vi "Excel_Read_XLSX.vi"(8 "error in (no error)":errorcluster, 10 "Truncate? (T)":bool=TRUE, 11 "Path in (xlsx,tsv,txt,csv,xml)":path) -> (0 "error out":errorcluster, 2 "Worksheets":T1(array[cluster]), 3 "Path out":path)   [LabVIEW 2018]
uses:
  <vilib>/zip/NI_Unzip.lvlib
  <vilib>/ErrorRing/Error Ring.xnode
  <vilib>/Utility/error.llb/Error Cluster From Error Code.vi
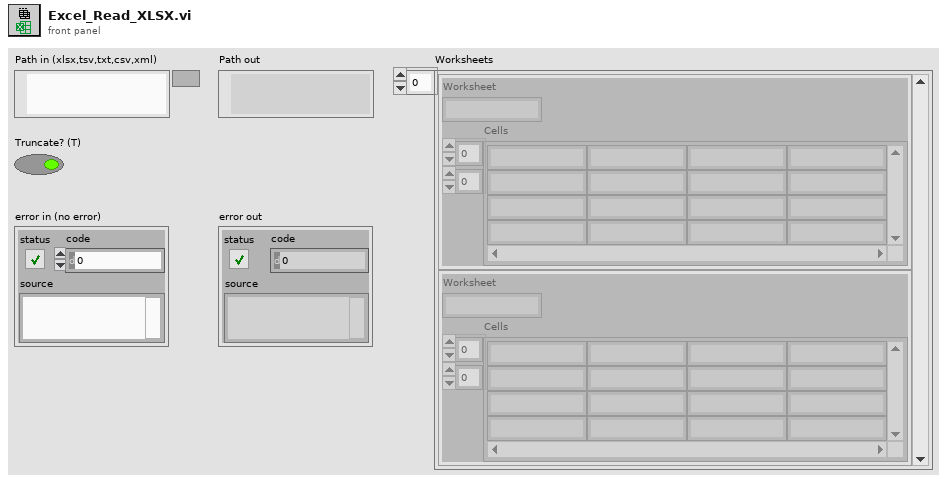
[diagram p1: front panel]
types:
  T1 = cluster{"Worksheet":string, "Cells":string[][]}[]
  T2 = cluster{"path":path, "sharedStrings.xml":string, "workbook.xml":string, "worksheet.xml":string[], "worksheet.xml IDs":i32[], "sharedStrings":string[], "SheetIDs":i32[], "Worksheets":cluster{"Worksheet":string, "Cells":string[][]}[], "sheetData":string[]}
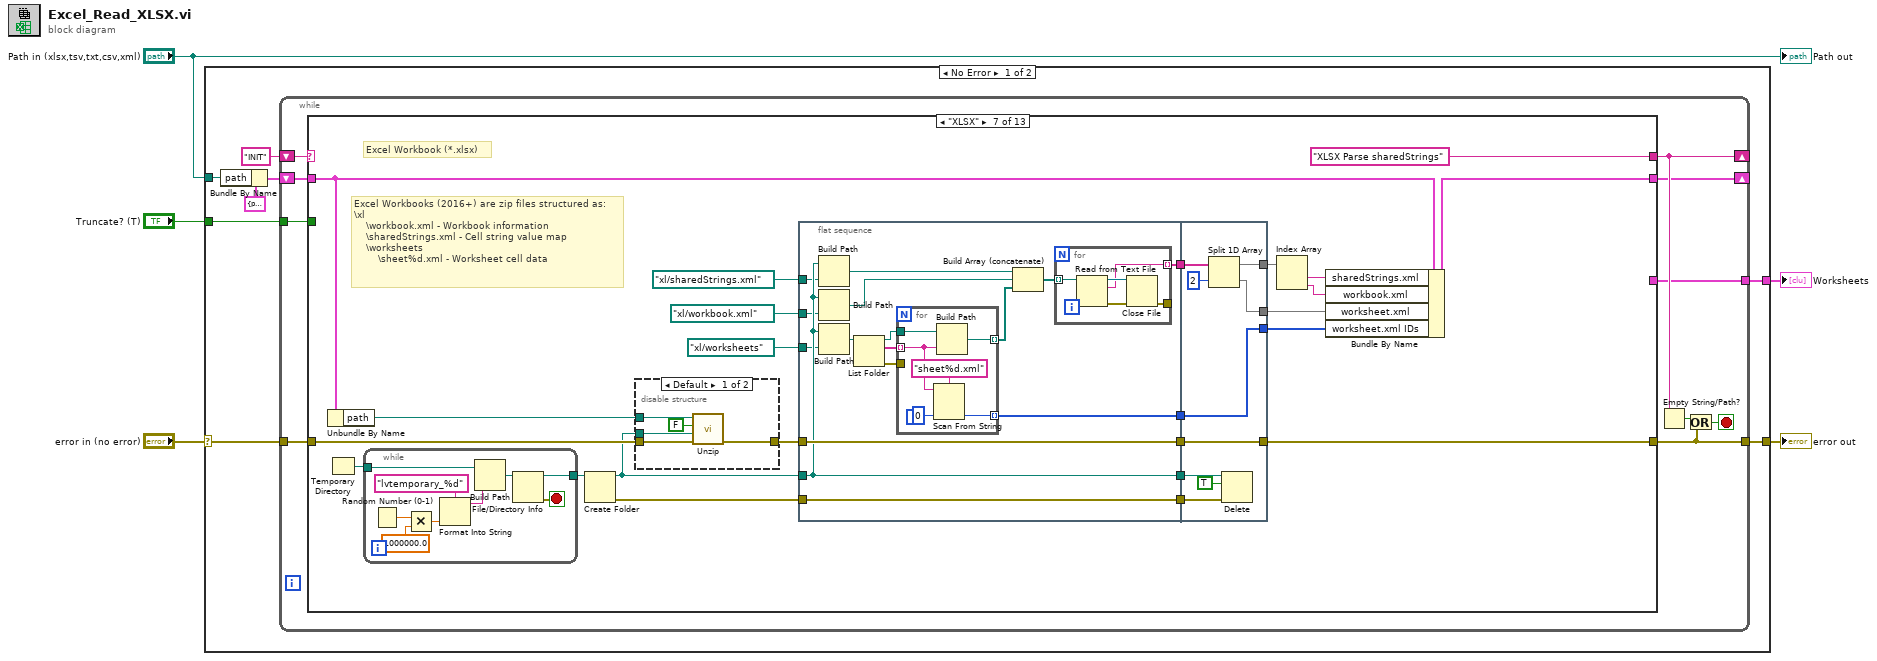
[diagram p0: block diagram]
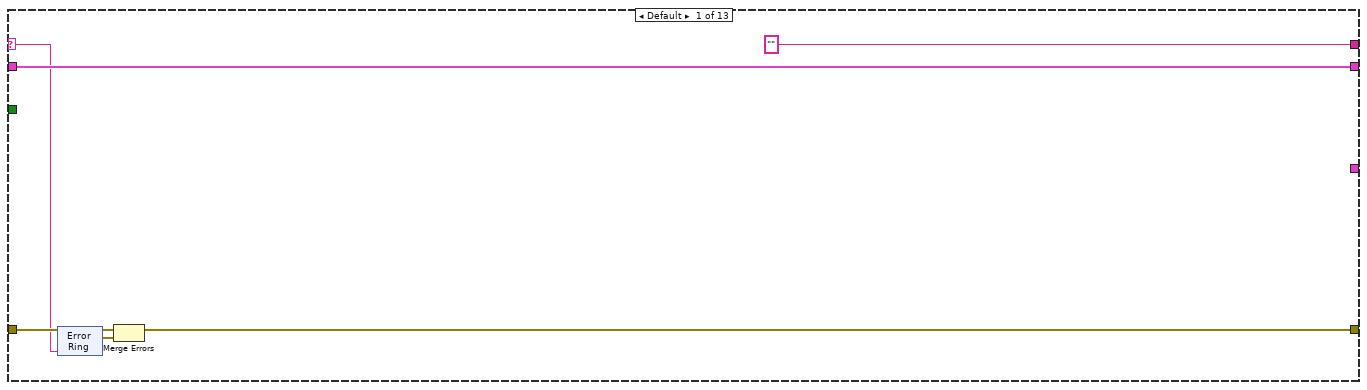
[diagram p2: hidden frame]
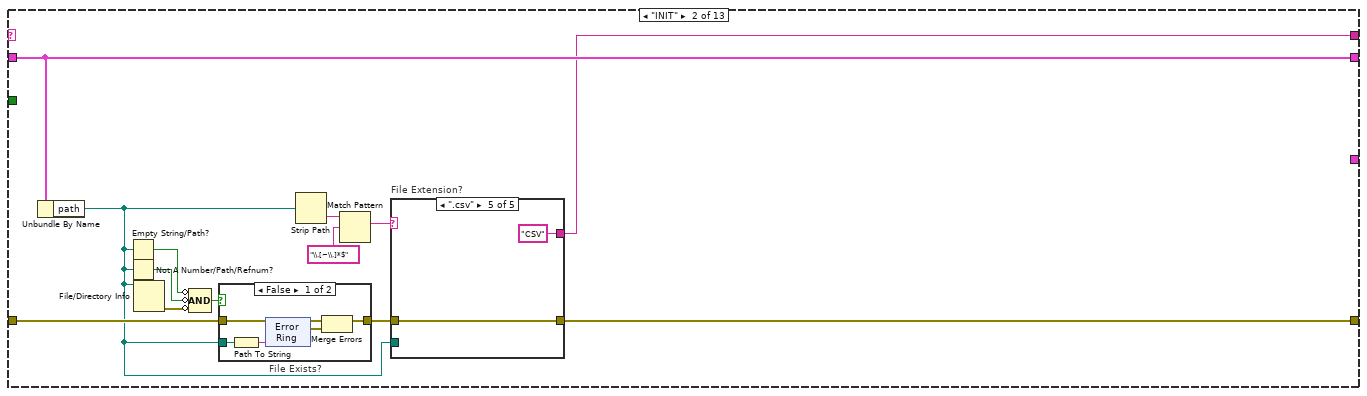
[diagram p3: hidden frame]
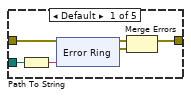
[diagram p4: hidden frame]
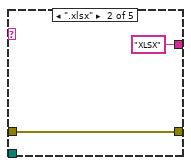
[diagram p5: hidden frame]
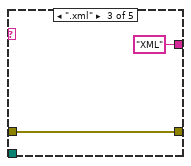
[diagram p6: hidden frame]
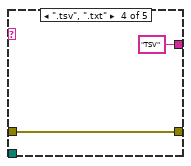
[diagram p7: hidden frame]
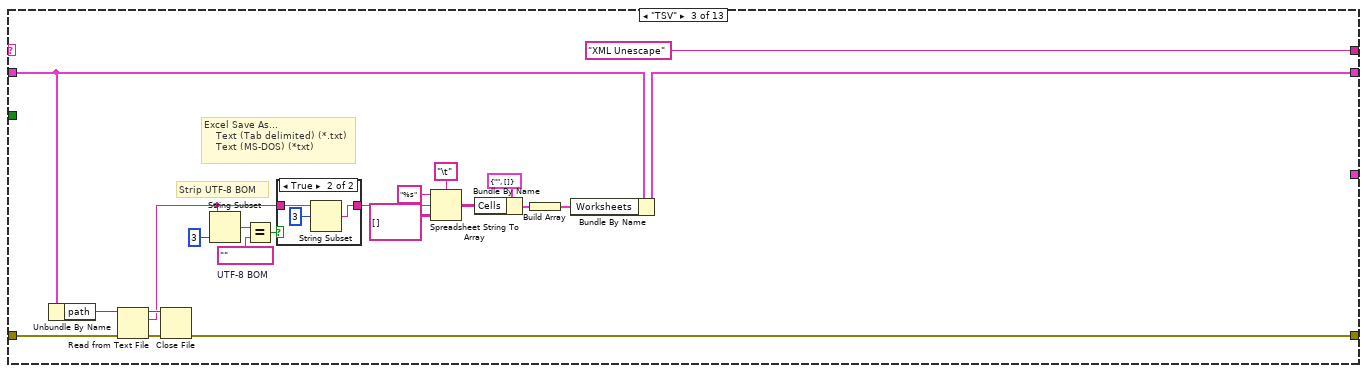
[diagram p9: hidden frame]
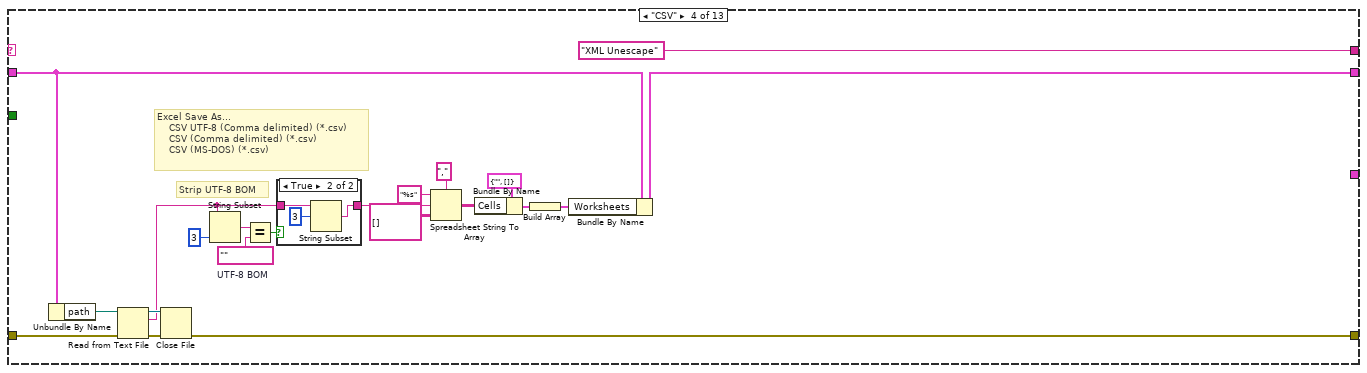
[diagram p11: hidden frame]
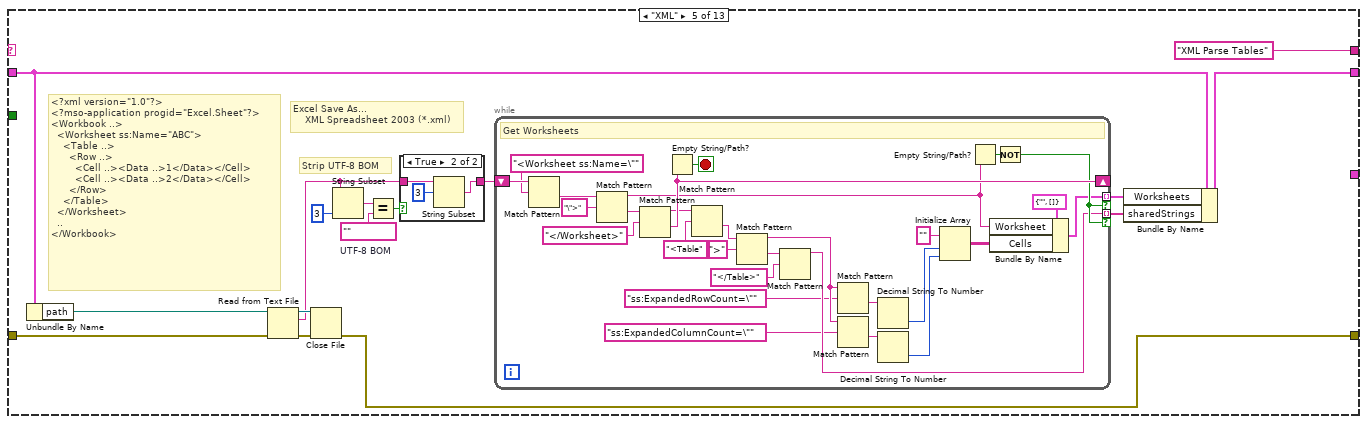
[diagram p13: hidden frame]
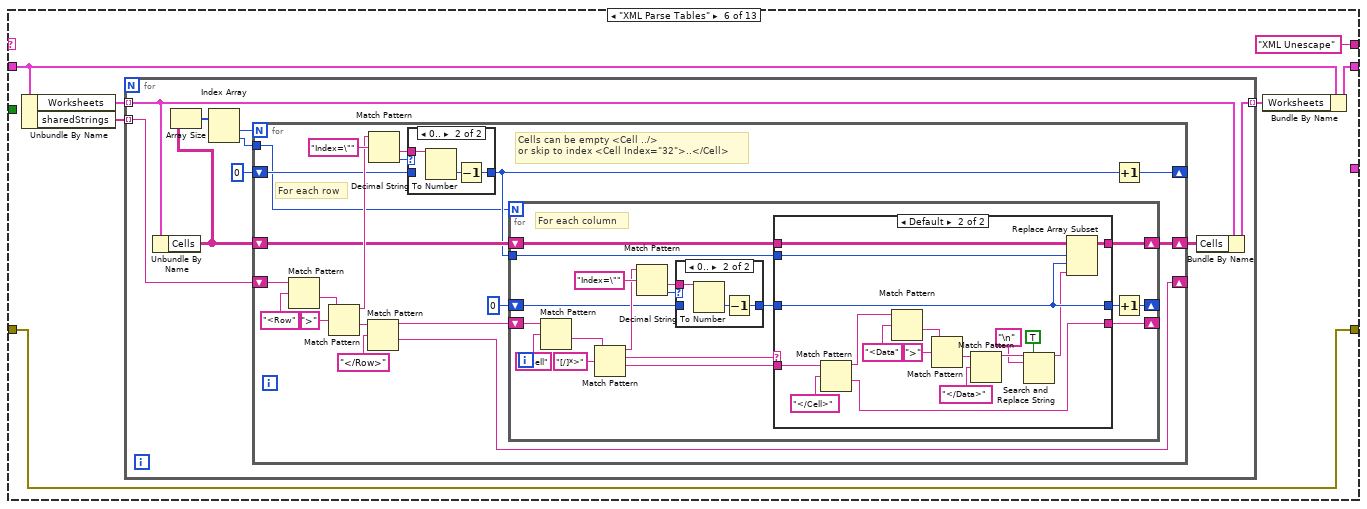
[diagram p15: hidden frame]
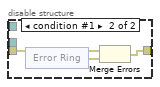
[diagram p19: hidden frame]
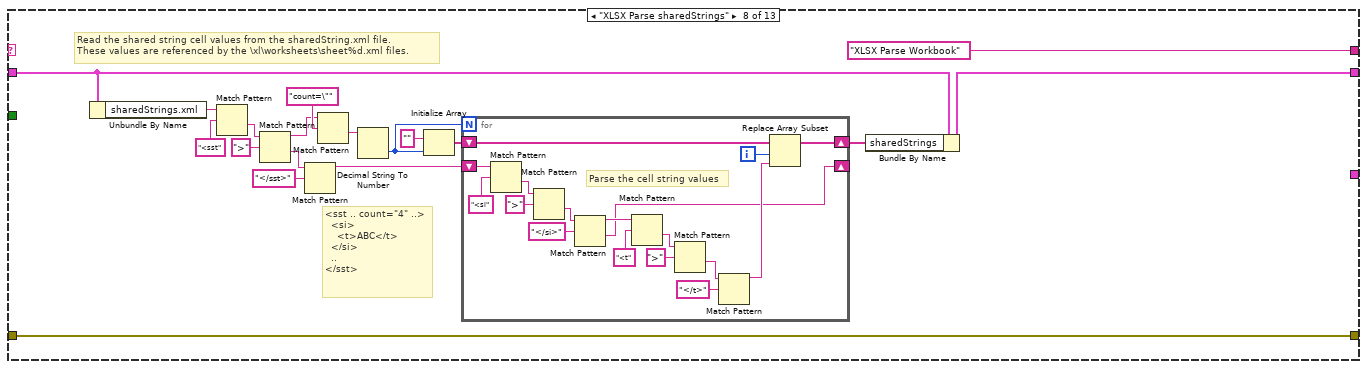
[diagram p20: hidden frame]
diagram:
  n1 = case shown="No Error" "error in (no error)" {
    selector: "error in (no error)" -> [w12 w624]
    tunnel: "Path in (xlsx,tsv,txt,csv,xml)" -> [w9 _]
    tunnel: [w8 w624] -> w3
    tunnel: [w7 _] -> w2
    tunnel: "Truncate? (T)" -> [w6 _]
    frame No Error {
      n2 = Bundle By Name(cluster=T2 {"path"=path "", "sharedStrings.xml"="", "workbook.xml"="", "worksheet.xml"=[], "worksheet.xml IDs"=[], "sharedStrings"=[], "SheetIDs"=[], "Worksheets"=[], "sheetData"=[]} ("StateData"), "path"=w9) -> (w10:T2)
      n3 = while {
        shift-right: [w18] -> _
        shift-left: "INIT" -> [w23]
        tunnel: w12 -> [w22]
        shift-right: [w16] -> _
        shift-left: w10 -> [w21]
        tunnel: [w20] -> w8
        tunnel: [w15] -> w7
        tunnel: w6 -> [w14]
        stop <- w19 stop-if-true
        n4 = case shown="\"XLSX\"" w23 {
          selector: w23 -> [w25 _ _ _ _ _ _ _ _ _ _ _ _]
          tunnel: w22 -> [w26 w46 w103 w128 w148 w187 w275 w345 w397 w431 w472 w551 w583]
          tunnel: w21 -> [w29 w44 w87 w113 w145 w188 w273 w362 w398 w432 w478 w554 w585]
          tunnel: [w27 w41 w90 w116 w133 w187 w274 w345 w397 w431 w472 w551 w583] -> w20
          tunnel: [w29 w44 w84 w109 w142 w186 w271 w349 w390 w429 w476 w550 w585] -> w16
          tunnel: ["" w38 "XML Unescape" "XML Unescape" "XML Parse Tables" "XML Unescape" "XLSX Parse sharedStrings" "XLSX Parse Workbook" "XLSX Parse Worksheets" "XLSX Parse sheetData" "XML Unescape" "Return Worksheets" _] -> w18
          tunnel: [_ _ _ _ _ _ _ _ _ _ _ _ w581] -> w15
          tunnel: w14 -> [_ _ _ _ _ _ _ _ _ _ _ _ w582]
          frame Default {
            n5 = xnode "Error Ring"("parameter 0"=w25) -> ("error out"=w28:errorcluster)
            n6 = Merge Errors(w26, w28) -> (w27:errorcluster)
          }
          frame "INIT" {
            n7 = Unbundle By Name(w44) -> ("path"=w37:path)
            n8 = Empty String/Path?(string/path=w37) -> (empty?=w48:bool)
            n9 = Not A Number/Path/Refnum?(number/path/refnum=w37) -> (NaN/Path/Refnum?=w49:bool)
            n10 = File/Directory Info(path=w37) -> (error out=w47:errorcluster)  [unwired: 1 in, 6 out]
            n11 = Compound Arithmetic op=AND(invert w48, invert w49, invert w47) -> (w45:bool)
            n12 = case "File Exists?" shown="False" w45 {
              tunnel: w46 -> [w72 w82]
              tunnel: w37 -> [w71 _]
              tunnel: [w70 w82] -> w40
              frame False {
                n13 = Path To String(path=w71) -> (string=w73:string)
                n14 = xnode "Error Ring"("parameter 0"=w73) -> ("error out"=w74:errorcluster)
                n15 = Merge Errors(w72, w74) -> (w70:errorcluster)
              }
              frame True {
              }
            }
            n16 = Strip Path(path=w37) -> (name=w43:string)  [unwired: 1 out]
            n17 = Match Pattern(string=w43, regular expression="\\.[~\\.]*$") -> (match substring=w39:string)  [unwired: 4 out]
            n18 = case "File Extension?" shown="\".csv\"" w39 {
              tunnel: [w52 w63 w65 w67 w69] -> w41
              tunnel: w40 -> [w53 w63 w65 w67 w69]
              tunnel: [_ "XLSX" "XML" "TSV" "CSV"] -> w38
              tunnel: w37 -> [w50 _ _ _ _]
              frame Default {
                n19 = Path To String(path=w50) -> (string=w51:string)
                n20 = xnode "Error Ring"("parameter 0"=w51) -> ("error out"=w54:errorcluster)
                n21 = Merge Errors(w53, w54) -> (w52:errorcluster)
              }
              frame ".xlsx" {
              }
              frame ".xml" {
              }
              frame ".tsv", ".txt" {
              }
              frame ".csv" {
              }
            }
          }
          frame "TSV" {
            w94 = "﻿"  # UTF-8 BOM
            # "Excel Save As...\n    Text (Tab delimited) (*.txt)\n    Text (MS-DOS) (*txt)"
            # "Strip UTF-8 BOM"
            n22 = Unbundle By Name(w87) -> ("path"=w86:path)
            n23 = Read from Text File(file (use dialog)=w86, error in=w103) -> (refnum out=w89:refnum<file>, text=w88:string, error out=w91:errorcluster)  [unwired: 2 in, 1 out]
            n24 = Close File(refnum=w89, error in=w91) -> (error out=w90:errorcluster)  [unwired: 1 out]
            n25 = String Subset(string=w88, length (rest)=3 ("length (rest)")) -> (substring=w95:string)  [unwired: 1 in]
            n26 = Equal?(x=w95, y=w94) -> (x = y?=w93:bool)
            n27 = case shown="True" w93 {
              tunnel: [w104 w107] -> w96
              tunnel: w88 -> [w104 w106]
              frame False {
              }
              frame True {
                n28 = String Subset(string=w106, offset (0)=3) -> (substring=w107:string)  [unwired: 1 in]
              }
            }
            n29 = Spreadsheet String To Array(delimiter (Tab)="\t", format string="%s", spreadsheet string=w96, array type (2D Dbl)=string[][] []) -> (array=w99:string[][])
            n30 = Bundle By Name(cluster=cluster{"Worksheet":string, "Cells":string[][]} {"Worksheet"="", "Cells"=[]}, "Cells"=w99) -> (w98:cluster{"Worksheet":string, "Cells":string[][]})
            n31 = Build Array(w98) -> (w83:T1)
            n32 = Bundle By Name(cluster=w87, "Worksheets"=w83) -> (w84:T2)
          }
          frame "CSV" {
            w119 = "﻿"  # UTF-8 BOM
            # "Excel Save As...\n    CSV UTF-8 (Comma delimited) (*.csv)\n    CSV (Comma delimited) (*.csv)\n    CSV (MS-DOS) (*.csv)"
            # "Strip UTF-8 BOM"
            n33 = Unbundle By Name(w113) -> ("path"=w112:path)
            n34 = Read from Text File(file (use dialog)=w112, error in=w128) -> (refnum out=w115:refnum<file>, text=w114:string, error out=w117:errorcluster)  [unwired: 2 in, 1 out]
            n35 = Close File(refnum=w115, error in=w117) -> (error out=w116:errorcluster)  [unwired: 1 out]
            n36 = String Subset(string=w114, length (rest)=3 ("length (rest)")) -> (substring=w120:string)  [unwired: 1 in]
            n37 = Equal?(x=w120, y=w119) -> (x = y?=w118:bool)
            n38 = case shown="True" w118 {
              tunnel: [w129 w132] -> w121
              tunnel: w114 -> [w129 w131]
              frame False {
              }
              frame True {
                n39 = String Subset(string=w131, offset (0)=3) -> (substring=w132:string)  [unwired: 1 in]
              }
            }
            n40 = Spreadsheet String To Array(delimiter (Tab)=",", format string="%s", spreadsheet string=w121, array type (2D Dbl)=string[][] []) -> (array=w124:string[][])
            n41 = Bundle By Name(cluster=cluster{"Worksheet":string, "Cells":string[][]} {"Worksheet"="", "Cells"=[]}, "Cells"=w124) -> (w123:cluster{"Worksheet":string, "Cells":string[][]})
            n42 = Build Array(w123) -> (w108:T1)
            n43 = Bundle By Name(cluster=w113, "Worksheets"=w108) -> (w109:T2)
          }
          frame "XML" {
            w139 = "﻿"  # UTF-8 BOM
            # "<?xml version=\"1.0\"?>\n<?mso-application progid=\"Excel.Sheet\"?>\n<Workbook ..>\n  <Worksheet ss:Name=\"ABC\">\n    <Table ..>\n      <Row ..>\n        <Cell ..><Data ..>1</Data></Cell>\n        <Cell ..><Data ..>2</Data></Cell>\n      </Row>\n    </Table>\n  </Worksheet>\n  ..\n</Workbook>"
            # "Excel Save As...\n    XML Spreadsheet 2003 (*.xml)"
            # "Strip UTF-8 BOM"
            n44 = Unbundle By Name(w145) -> ("path"=w144:path)
            n45 = Read from Text File(file (use dialog)=w144, error in=w148) -> (refnum out=w146:refnum<file>, text=w136:string, error out=w147:errorcluster)  [unwired: 2 in, 1 out]
            n46 = Close File(refnum=w146, error in=w147) -> (error out=w133:errorcluster)  [unwired: 1 out]
            n47 = String Subset(string=w136, length (rest)=3 ("length (rest)")) -> (substring=w138:string)  [unwired: 1 in]
            n48 = Equal?(x=w138, y=w139) -> (x = y?=w140:bool)
            n49 = case shown="True" w140 {
              tunnel: [w178 w181] -> w141
              tunnel: w136 -> [w178 w180]
              frame False {
              }
              frame True {
                n50 = String Subset(string=w180, offset (0)=3) -> (substring=w181:string)  [unwired: 1 in]
              }
            }
            n51 = while {
              shift-right: [w171] -> _
              shift-left: w141 -> [w177]
              tunnel: [w165] -> w134 mode=indexing if=w168
              tunnel: [w157] -> w135 mode=indexing if=w168
              stop <- w170 stop-if-true
              # "Get Worksheets"
              n52 = Match Pattern(string=w177, regular expression="<Worksheet ss:Name=\"") -> (after substring=w175:string)  [unwired: 1 in, 3 out]
              n53 = Match Pattern(string=w175, regular expression="\">") -> (before substring=w166:string, after substring=w172:string)  [unwired: 1 in, 2 out]
              n54 = Match Pattern(string=w172, regular expression="</Worksheet>") -> (before substring=w158:string, after substring=w171:string)  [unwired: 1 in, 2 out]
              n55 = Empty String/Path?(string/path=w171) -> (empty?=w170:bool)
              n56 = Match Pattern(string=w158, regular expression="<Table") -> (after substring=w161:string)  [unwired: 1 in, 3 out]
              n57 = Match Pattern(string=w161, regular expression=">") -> (before substring=w152:string, after substring=w164:string)  [unwired: 1 in, 2 out]
              n58 = Match Pattern(string=w164, regular expression="</Table>") -> (before substring=w157:string)  [unwired: 1 in, 3 out]
              n59 = Match Pattern(string=w152, regular expression="ss:ExpandedRowCount=\"") -> (after substring=w153:string)  [unwired: 1 in, 3 out]
              n60 = Match Pattern(string=w152, regular expression="ss:ExpandedColumnCount=\"") -> (after substring=w155:string)  [unwired: 1 in, 3 out]
              n61 = Decimal String To Number(string=w153) -> (number=w150:i32)  [unwired: 2 in, 1 out]
              n62 = Decimal String To Number(string=w155) -> (number=w154:i32)  [unwired: 2 in, 1 out]
              n63 = Initialize Array("", w150, w154) -> (w149:string[][])
              n64 = Empty String/Path?(string/path=w166) -> (empty?=w169:bool)
              n65 = Bundle By Name(cluster=cluster{"Worksheet":string, "Cells":string[][]} {"Worksheet"="", "Cells"=[]}, "Worksheet"=w166, "Cells"=w149) -> (w165:cluster{"Worksheet":string, "Cells":string[][]})
              n66 = Not(x=w169) -> (.not. x?=w168:bool)
            }
            n67 = Bundle By Name(cluster=w145, "Worksheets"=w134, "sharedStrings"=w135) -> (w142:T2)
          }
          frame "XML Parse Tables" {
            n68 = Unbundle By Name(w188) -> ("Worksheets"=w185:T1, "sharedStrings"=w184:string[])
            n69 = for {
              tunnel: w185 -> [w195] mode=indexing
              tunnel: w184 -> [w196] mode=indexing
              tunnel: [w190] -> w183 mode=indexing
              n70 = Unbundle By Name(w195) -> ("Cells"=w191:string[][])
              n71 = Array Size(array=w191) -> (size(s)=w194:i32[])
              n72 = Index Array(array=w194) -> (element #1=w193:i32, element #2=w192:i32)  [unwired: 2 in]
              n73 = for {
                N: w193 -> [_]
                shift-right: [w207] -> w189
                shift-left: w191 -> [w206]
                shift-right: [w204] -> _
                shift-left: 0 -> [w209]
                shift-right: [w200] -> _
                shift-left: w196 -> [w216]
                tunnel: w192 -> [w198]
                # "Cells can be empty <Cell ../>\nor skip to index <Cell Index=\"32\">..</Cell>"
                # "For each row"
                n74 = Match Pattern(string=w216, regular expression="<Row") -> (after substring=w213:string)  [unwired: 1 in, 3 out]
                n75 = Match Pattern(string=w213, regular expression=">") -> (before substring=w211:string, after substring=w202:string)  [unwired: 1 in, 2 out]
                n76 = Match Pattern(string=w202, regular expression="</Row>") -> (before substring=w201:string, after substring=w200:string)  [unwired: 1 in, 2 out]
                n77 = Match Pattern(string=w211, regular expression="Index=\"") -> (after substring=w210:string, offset past match=w208:i32)  [unwired: 1 in, 2 out]
                n78 = case shown="0.." w208 {
                  tunnel: w210 -> [_ w262]
                  tunnel: w209 -> [w259 _]
                  tunnel: [w259 w260] -> w205
                  frame ..-1 {
                  }
                  frame 0.. {
                    n79 = Decimal String To Number(string=w262) -> (number=w261:i32)  [unwired: 2 in, 1 out]
                    n80 = Decrement(x=w261) -> (x-1=w260:i32)
                  }
                }
                n81 = for {
                  N: w198 -> [_]
                  shift-right: [w233] -> w207
                  shift-left: w206 -> [w234]
                  tunnel: w205 -> [w232]
                  shift-right: [w221] -> _
                  shift-left: 0 -> [w220]
                  shift-right: [w217] -> _
                  shift-left: w201 -> [w227]
                  # "For each column"
                  n82 = Match Pattern(string=w227, regular expression="<Cell") -> (after substring=w230:string)  [unwired: 1 in, 3 out]
                  n83 = Match Pattern(string=w230, regular expression="[/]*>") -> (before substring=w223:string, match substring=w219:string, after substring=w231:string)  [unwired: 1 in, 1 out]
                  n84 = Match Pattern(string=w223, regular expression="Index=\"") -> (after substring=w225:string, offset past match=w226:i32)  [unwired: 1 in, 2 out]
                  n85 = case shown="0.." w226 {
                    tunnel: w225 -> [_ w258]
                    tunnel: w220 -> [w255 _]
                    tunnel: [w255 w256] -> w222
                    frame ..-1 {
                    }
                    frame 0.. {
                      n86 = Decimal String To Number(string=w258) -> (number=w257:i32)  [unwired: 2 in, 1 out]
                      n87 = Decrement(x=w257) -> (x-1=w256:i32)
                    }
                  }
                  n88 = case shown="Default" w219 {
                    tunnel: w234 -> [w237 w254]
                    tunnel: [w237 w253] -> w233
                    tunnel: w232 -> [_ w252]
                    tunnel: w231 -> [w235 w251]
                    tunnel: w222 -> [w236 w249]
                    tunnel: [w236 w249] -> w218
                    tunnel: [w235 w242] -> w217
                    frame "/>" {
                      # "No cell data"
                    }
                    frame Default {
                      n89 = Match Pattern(string=w251, regular expression="</Cell>") -> (before substring=w243:string, after substring=w242:string)  [unwired: 1 in, 2 out]
                      n90 = Match Pattern(string=w243, regular expression="<Data") -> (after substring=w246:string)  [unwired: 1 in, 3 out]
                      n91 = Match Pattern(string=w246, regular expression=">") -> (after substring=w248:string)  [unwired: 1 in, 3 out]
                      n92 = Match Pattern(string=w248, regular expression="</Data>") -> (before substring=w241:string)  [unwired: 1 in, 3 out]
                      n93 = Search and Replace String(replace all?=TRUE ("replace all? (F)"), input string=w241, search string="\n") -> (result string=w240:string)  [unwired: 5 in, 3 out]
                      n94 = Replace Array Subset(array=w254, new element=w240, index (row)=w252, index (col)=w249) -> (w253:string[][])
                    }
                  }
                  n95 = Increment(x=w218) -> (x+1=w221:i32)
                }
                n96 = Increment(x=w205) -> (x+1=w204:i32)
              }
              n97 = Bundle By Name(cluster=w195, "Cells"=w189) -> (w190:cluster{"Worksheet":string, "Cells":string[][]})
            }
            n98 = Bundle By Name(cluster=w188, "Worksheets"=w183) -> (w186:T2)
          }
          frame "XLSX" {
            # "Excel Workbook (*.xlsx)"
            # "Excel Workbooks (2016+) are zip files structured as:\n\\xl\n    \\workbook.xml - Workbook information\n    \\sharedStrings.xml - Cell string value map\n    \\worksheets\n        \\sheet%d.xml - Worksheet cell data"
            n99 = Unbundle By Name(w273) -> ("path"=w272:path)
            n100 = Temporary Directory() -> (w282:path)
            n101 = while {
              tunnel: [w337] -> w279
              tunnel: w282 -> [w336]
              stop <- w338 stop-if-true
              n102 = Random Number (0-1)() -> (number: 0 to 1=w344:dbl)
              n103 = Multiply(x=w344, y=1000000.0) -> (x*y=w341:dbl)
              n104 = Format Into String(format string="lvtemporary_%d", w341) -> (resulting string=w340:string)  [unwired: 2 in, 1 out]
              n105 = Build Path(base path=w336, name or relative path=w340) -> (appended path=w339:path)
              n106 = File/Directory Info(path=w339) -> (path out=w337:path, error out=w338:errorcluster)  [unwired: 1 in, 5 out]
            }
            n107 = Create Folder(path (use dialog)=w279) -> (created path=w269:path, error out=w281:errorcluster)  [unwired: 2 in, 1 out]
            n108 = disable-structure shown="Default" {
              disable-tunnel: [w291 w293] -> w280
              disable-tunnel: w275 -> [w289 w294]
              disable-tunnel: w272 -> [w288 _]
              disable-tunnel: w269 -> [w287 _]
              frame condition #0 (active) {
                n109 = call <vilib>:"Unzip.vi"("error in (no error)"=w289, "Target directory (same as Zip file if empty)"=w287, "Preview only?"=FALSE, "Zip file"=w288) -> ("error out"=w291:errorcluster)  [unwired: 5 in, 2 out]
              }
              frame condition #1 {
                n110 = xnode "Error Ring"() -> ("error out"=w292:errorcluster)
                n111 = Merge Errors(w294, w292) -> (w293:errorcluster)
              }
            }
            n112 = flat-sequence {
              tunnel: w269 -> [w308]
              tunnel: w280 -> [w309]
              tunnel: [w309] -> w286
              tunnel: [w308] -> w285
              tunnel: w281 -> [w307]
              tunnel: [w307] -> w284
              tunnel: [w306] -> w283
              tunnel: path "xl/worksheets" ("name or relative path") -> [w304]
              tunnel: path "xl/sharedStrings.xml" ("name or relative path") -> [w303]
              tunnel: path "xl/workbook.xml" ("name or relative path") -> [w302]
              tunnel: [w300] -> w267
              tunnel: [w335] -> w274
              tunnel: w286 -> [w335]
              tunnel: w285 -> [w334]
              tunnel: w284 -> [w332]
              tunnel: w283 -> [w330]
              tunnel: [w331] -> w268
              tunnel: w267 -> [w331]
              tunnel: [w328] -> w266
              tunnel: [w327] -> w263
              frame #0 {
                n113 = Build Path(base path=w308, name or relative path=w303) -> (appended path=w313:path)
                n114 = Build Path(base path=w308, name or relative path=w302) -> (appended path=w312:path)
                n115 = Build Path(base path=w308, name or relative path=w304) -> (appended path=w315:path)
                n116 = List Folder(path=w315) -> (path out=w314:path, filenames=w301:string[], error out=w305:errorcluster)  [unwired: 3 in, 1 out]
                n117 = for {
                  tunnel: w314 -> [w326]
                  tunnel: w301 -> [w324] mode=indexing
                  tunnel: [w325] -> w311 mode=indexing
                  tunnel: w305 -> [_]
                  tunnel: [w321] -> w300 mode=indexing
                  n118 = Scan From String(format string="sheet%d.xml", input string=w324, default 1=0 ("default value 1")) -> (output 1=w321:i32)  [unwired: 2 in, 3 out]
                  n119 = Build Path(base path=w326, name or relative path=w324) -> (appended path=w325:path)
                }
                n120 = Build Array (concatenate)(w313, w312, w311) -> (w310:path[])
                n121 = for {
                  tunnel: w310 -> [w318] mode=indexing
                  tunnel: [w317] -> w306 mode=indexing
                  tunnel: [w316] -> _
                  n122 = Read from Text File(file (use dialog)=w318) -> (refnum out=w320:refnum<file>, text=w317:string, error out=w319:errorcluster)  [unwired: 3 in, 1 out]
                  n123 = Close File(refnum=w320, error in=w319) -> (error out=w316:errorcluster)  [unwired: 1 out]
                }
              }
              frame #1 {
                n124 = Split 1D Array(array=w330, index=2) -> (first subarray=w328:string[], second subarray=w327:string[])
                n125 = Delete(path (use dialog)=w334, entire hierarchy (F)=TRUE, error in=w332) -> ()  [unwired: 2 in, 3 out]
              }
            }
            n126 = Index Array(array=w266) -> (element #1=w265:string, element #2=w264:string)  [unwired: 2 in]
            n127 = Bundle By Name(cluster=w273, "sharedStrings.xml"=w265, "workbook.xml"=w264, "worksheet.xml"=w263, "worksheet.xml IDs"=w268) -> (w271:T2)
          }
          frame "XLSX Parse sharedStrings" {
            # "Read the shared string cell values from the sharedString.xml file.\nThese values are referenced by the \\xl\\worksheets\\sheet%d.xml files."
            # "<sst .. count=\"4\" ..>\n  <si>\n    <t>ABC</t>\n  </si>\n  ..\n</sst>"
            n128 = Unbundle By Name(w362) -> ("sharedStrings.xml"=w361:string)
            n129 = Match Pattern(string=w361, regular expression="<sst") -> (after substring=w358:string)  [unwired: 1 in, 3 out]
            n130 = Match Pattern(string=w358, regular expression=">") -> (before substring=w356:string, after substring=w351:string)  [unwired: 1 in, 2 out]
            n131 = Match Pattern(string=w351, regular expression="</sst>") -> (before substring=w350:string)  [unwired: 1 in, 3 out]
            n132 = Match Pattern(string=w356, regular expression="count=\"") -> (after substring=w355:string)  [unwired: 1 in, 3 out]
            n133 = Decimal String To Number(string=w355) -> (number=w346:i32)  [unwired: 2 in, 1 out]
            n134 = Initialize Array("", w346) -> (w353:string[])
            n135 = for {
              N: w346 -> [_]
              shift-right: [w364] -> w348
              shift-left: w353 -> [w376]
              shift-right: [w363] -> _
              shift-left: w350 -> [w375]
              i -> [w366]
              # "Parse the cell string values"
              n136 = Match Pattern(string=w375, regular expression="<si") -> (after substring=w379:string)  [unwired: 1 in, 3 out]
              n137 = Match Pattern(string=w379, regular expression=">") -> (after substring=w370:string)  [unwired: 1 in, 3 out]
              n138 = Match Pattern(string=w370, regular expression="</si>") -> (before substring=w369:string, after substring=w363:string)  [unwired: 1 in, 2 out]
              n139 = Match Pattern(string=w369, regular expression="<t") -> (after substring=w372:string)  [unwired: 1 in, 3 out]
              n140 = Match Pattern(string=w372, regular expression=">") -> (after substring=w367:string)  [unwired: 1 in, 3 out]
              n141 = Match Pattern(string=w367, regular expression="</t>") -> (before substring=w365:string)  [unwired: 1 in, 3 out]
              n142 = Replace Array Subset(array=w376, new element=w365, index=w366) -> (w364:string[])
            }
            n143 = Bundle By Name(cluster=w362, "sharedStrings"=w348) -> (w349:T2)
          }
          frame "XLSX Parse Workbook" {
            # "The workbook.xml file contains the reference sheet IDs (r:id=\"rId%d\")\nneeded to load the correct \\xl\\worksheets\\sheet%d.xml files."
            # "<workbook ..>\n  <sheets ..>\n    <sheet name=\"Sheet1\" sheetId=\"1\" r:id=\"rId1\"/>\n  </sheets>\n</workbook>"
            n144 = Unbundle By Name(w398) -> ("workbook.xml"=w396:string)
            n145 = Match Pattern(string=w396, regular expression="<workbook") -> (after substring=w393:string)  [unwired: 1 in, 3 out]
            n146 = Match Pattern(string=w393, regular expression=">") -> (after substring=w391:string)  [unwired: 1 in, 3 out]
            n147 = Match Pattern(string=w391, regular expression="</workbook>") -> (before substring=w383:string)  [unwired: 1 in, 3 out]
            n148 = Match Pattern(string=w383, regular expression="<sheets") -> (after substring=w386:string)  [unwired: 1 in, 3 out]
            n149 = Match Pattern(string=w386, regular expression=">") -> (after substring=w388:string)  [unwired: 1 in, 3 out]
            n150 = Match Pattern(string=w388, regular expression="</sheets>") -> (before substring=w382:string)  [unwired: 1 in, 3 out]
            n151 = while {
              shift-right: [w412] -> _
              shift-left: w382 -> [w414]
              tunnel: [w401] -> w380 mode=indexing if=w399
              tunnel: [w400] -> w381 mode=indexing if=w399
              stop <- w411 stop-if-true
              # "Parse Sheet"
              n152 = Match Pattern(string=w414, regular expression="<sheet") -> (after substring=w415:string, offset past match=w413:i32)  [unwired: 1 in, 2 out]
              n153 = case shown="0.." w413 {
                tunnel: "[/]*>" ("regular expression") -> [_ w422]
                tunnel: w415 -> [_ w421]
                tunnel: [_ w420] -> w412
                tunnel: [_ w419] -> w406
                tunnel: [_ TRUE] -> w399
                frame ..-1 {
                }
                frame 0.. {
                  n154 = Match Pattern(string=w421, regular expression=w422) -> (before substring=w419:string, after substring=w420:string)  [unwired: 1 in, 2 out]
                }
              }
              n155 = Match Pattern(string=w406, regular expression="r:id=\"rId") -> (after substring=w405:string)  [unwired: 1 in, 3 out]
              n156 = Match Pattern(string=w406, regular expression="name=\"") -> (after substring=w408:string)  [unwired: 1 in, 3 out]
              n157 = Empty String/Path?(string/path=w412) -> (empty?=w411:bool)
              n158 = Decimal String To Number(string=w405, default (0L)=0 ("default (0 I32)")) -> (number=w400:i32)  [unwired: 1 in, 1 out]
              n159 = Match Pattern(string=w408, regular expression="\"") -> (before substring=w402:string)  [unwired: 1 in, 3 out]
              n160 = Bundle By Name(cluster=cluster{"Worksheet":string, "Cells":string[][]} {"Worksheet"="", "Cells"=[]}, "Worksheet"=w402) -> (w401:cluster{"Worksheet":string, "Cells":string[][]})
            }
            n161 = Bundle By Name(cluster=w398, "SheetIDs"=w381, "Worksheets"=w380) -> (w390:T2)
          }
          frame "XLSX Parse Worksheets" {
            # "Sheet%d.xml contain the sheet cell data, the dimension field specified the size of the worksheet."
            # "<worksheet ..>\n  <dimension ref=\"A1:C2\"/>\n  <sheetData ..>\n    <sheet name=\"Sheet1\" sheetId=\"1\" r:id=\"rId1\"/>\n  </sheetData>\n</worksheet>"
            n162 = Unbundle By Name(w432) -> ("Worksheets"=w424:T1, "worksheet.xml"=w430:string[], "worksheet.xml IDs"=w427:i32[], "SheetIDs"=w426:i32[])
            n163 = for {
              tunnel: w430 -> [w470]
              tunnel: w427 -> [w444]
              tunnel: w426 -> [w443] mode=indexing
              tunnel: [w440] -> w425 mode=indexing
              tunnel: w424 -> [w441] mode=indexing
              tunnel: [w438] -> w423 mode=indexing
              n164 = Search 1D Array(1D array=w444, element=w443) -> (index of element=w442:i32)  [unwired: 1 in]
              n165 = Index Array(array=w470, index=w442) -> (element=w455:string)
              n166 = Match Pattern(string=w455, regular expression="<worksheet") -> (after substring=w467:string)  [unwired: 1 in, 3 out]
              n167 = Match Pattern(string=w467, regular expression=">") -> (after substring=w465:string)  [unwired: 1 in, 3 out]
              n168 = Match Pattern(string=w465, regular expression="</worksheet>") -> (before substring=w456:string)  [unwired: 1 in, 3 out]
              n169 = Match Pattern(string=w456, regular expression="<dimension") -> (after substring=w457:string)  [unwired: 1 in, 3 out]
              n170 = Match Pattern(string=w456, regular expression="<sheetData") -> (after substring=w462:string)  [unwired: 1 in, 3 out]
              n171 = Match Pattern(string=w457, regular expression="[/]*>") -> (before substring=w453:string)  [unwired: 1 in, 3 out]
              n172 = Match Pattern(string=w462, regular expression=">") -> (after substring=w464:string)  [unwired: 1 in, 3 out]
              n173 = Match Pattern(string=w453, regular expression="ref=\"") -> (after substring=w452:string)  [unwired: 1 in, 3 out]
              n174 = Match Pattern(string=w464, regular expression="</sheetData>") -> (before substring=w438:string)  [unwired: 1 in, 3 out]
              n175 = Scan From String(format string="%[0-9A-Z]:%[0-9A-Z]\"", input string=w452) -> (output 1=w450:string, output 2=w437:string)  [unwired: 4 in, 3 out]
              n176 = call "Excel Cell to RowCol.vi"("Cell ([A-Z..][0-9..])"=w450) -> ("Column"=w448:i32, "Row"=w449:i32)  [unwired: 9 in]
              n177 = call "Excel Cell to RowCol.vi"("Cell ([A-Z..][0-9..])"=w437) -> ("Column"=w435:i32, "Row"=w436:i32)  [unwired: 9 in]
              n178 = Subtract(x=w436, y=w449) -> (x-y=w447:i32)
              n179 = Subtract(x=w435, y=w448) -> (x-y=w446:i32)
              n180 = Increment(x=w447) -> (x+1=w434:i32)
              n181 = Increment(x=w446) -> (x+1=w433:i32)
              n182 = Initialize Array("", w434, w433) -> (w439:string[][])
              n183 = Bundle By Name(cluster=w441, "Cells"=w439) -> (w440:cluster{"Worksheet":string, "Cells":string[][]})
            }
            n184 = Bundle By Name(cluster=w432, "Worksheets"=w425, "sheetData"=w423) -> (w429:T2)
          }
          frame "XLSX Parse sheetData" {
            # "The sheet%d.xml contains the 'sheetData' cells that contain the cell value or reference the '\\xl\\sharedStrings.xml' value map.\nKnown type attribute (t=\"x\"): b=Boolean, s=sharedStrings Reference, other==cell value"
            n185 = Unbundle By Name(w478) -> ("sharedStrings"=w471:string[], "Worksheets"=w473:T1, "sheetData"=w477:string[])
            n186 = for {
              tunnel: w477 -> [w484] mode=indexing
              tunnel: [w482] -> w474 mode=indexing
              tunnel: w473 -> [w483] mode=indexing
              tunnel: w471 -> [w479]
              n187 = Unbundle By Name(w483) -> ("Cells"=w481:string[][])
              n188 = while {
                shift-right: [w489] -> _
                shift-left: w484 -> [w490]
                shift-right: [w486] -> w480
                shift-left: w481 -> [w487]
                tunnel: w479 -> [w485]
                stop <- w488 stop-if-true
                # "<row r=\"1\" spans=\"1:3\" ..>\n  <c r=\"A1\" t=\"s\">\n    <v>0</v>\n  </c>\n  <c r=\"B1\" .. />\n  ..\n</row>"
                n189 = Match Pattern(string=w490, regular expression="<row") -> (after substring=w494:string)  [unwired: 1 in, 3 out]
                n190 = Match Pattern(string=w494, regular expression=">") -> (after substring=w492:string)  [unwired: 1 in, 3 out]
                n191 = Match Pattern(string=w492, regular expression="</row>") -> (before substring=w491:string, after substring=w489:string)  [unwired: 1 in, 2 out]
                n192 = while {
                  shift-right: [w500] -> _
                  shift-left: w491 -> [w504]
                  shift-right: [w502] -> w486
                  shift-left: w487 -> [w503]
                  tunnel: w485 -> [w498]
                  stop <- w499 stop-if-true
                  n193 = Match Pattern(string=w504, regular expression="<c") -> (after substring=w507:string)  [unwired: 1 in, 3 out]
                  n194 = Match Pattern(string=w507, regular expression="[/]*>") -> (before substring=w501:string, match substring=w497:string, after substring=w508:string)  [unwired: 1 in, 1 out]
                  n195 = case shown="Default" w497 {
                    tunnel: w508 -> [w509 w537]
                    tunnel: w503 -> [w510 w530]
                    tunnel: [w510 w527] -> w502
                    tunnel: w501 -> [_ w525]
                    tunnel: [w509 w522] -> w500
                    tunnel: w498 -> [_ w519]
                    frame "/>" {
                    }
                    frame Default {
                      n196 = Match Pattern(string=w525, regular expression="r=\"") -> (after substring=w535:string)  [unwired: 1 in, 3 out]
                      n197 = Match Pattern(string=w525, regular expression="t=\"") -> (after substring=w524:string)  [unwired: 1 in, 3 out]
                      n198 = Match Pattern(string=w537, regular expression="</c>") -> (before substring=w511:string, after substring=w522:string)  [unwired: 1 in, 2 out]
                      n199 = Match Pattern(string=w524, regular expression="\"") -> (before substring=w520:string)  [unwired: 1 in, 3 out]
                      n200 = Scan From String(format string="%[0-9A-Z]\"", input string=w535) -> (output 1=w533:string)  [unwired: 3 in, 3 out]
                      n201 = Match Pattern(string=w511, regular expression="<v") -> (after substring=w514:string)  [unwired: 1 in, 3 out]
                      n202 = Match Pattern(string=w514, regular expression=">") -> (after substring=w512:string)  [unwired: 1 in, 3 out]
                      n203 = call "Excel Cell to RowCol.vi"("Cell ([A-Z..][0-9..])"=w533) -> ("Column"=w531:i32, "Row"=w532:i32)  [unwired: 9 in]
                      n204 = Match Pattern(string=w512, regular expression="</v>") -> (before substring=w521:string)  [unwired: 1 in, 3 out]
                      n205 = Decrement(x=w532) -> (x-1=w529:i32)
                      n206 = Decrement(x=w531) -> (x-1=w528:i32)
                      n207 = case "Type" shown="\"s\"" w520 {
                        tunnel: w521 -> [w538 w543 w545]
                        tunnel: w519 -> [_ w540 _]
                        tunnel: [w538 w539 w544] -> w518
                        frame Default {
                        }
                        frame "s" {
                          n208 = Decimal String To Number(string=w543, default (0L)=-1 ("default (0 I32)")) -> (number=w541:i32)  [unwired: 1 in, 1 out]
                          n209 = Index Array(array=w540, index=w541) -> (element=w539:string)
                        }
                        frame "b" {
                          n210 = case shown="\"0\", Default" w545 {
                            tunnel: ["FALSE" "TRUE"] -> w544
                            frame "0", Default {
                            }
                            frame "1" {
                            }
                          }
                        }
                      }
                      n211 = Replace Array Subset(array=w530, new element=w518, index (row)=w529, index (col)=w528) -> (w527:string[][])
                    }
                  }
                  n212 = Empty String/Path?(string/path=w500) -> (empty?=w499:bool)
                }
                n213 = Empty String/Path?(string/path=w489) -> (empty?=w488:bool)
              }
              n214 = Bundle By Name(cluster=w483, "Cells"=w480) -> (w482:cluster{"Worksheet":string, "Cells":string[][]})
            }
            n215 = Bundle By Name(cluster=w478, "Worksheets"=w474) -> (w476:T2)
          }
          frame "XML Unescape" {
            n216 = Unbundle By Name(w554) -> ("Worksheets"=w552:T1)
            n217 = for {
              tunnel: string[][] [["&amp;", "&"], ["&lt;", "<"], ["&gt;", ">"], ["&apos;", "'"], ["&quot;", "\""]] -> [w557]
              tunnel: w552 -> [w556] mode=indexing
              tunnel: [w555] -> w549 mode=indexing
              n218 = in-place {
                in-place-border: w557 -> [w558]
                n219 = in-place-cluster #1(w556) -> ("Worksheet"=w562:string, "Cells"=w560:string[][])
                n220 = for {
                  shift-right: [w578] -> w561
                  shift-left: w562 -> [w580]
                  tunnel: w558 -> [w577] mode=indexing
                  n221 = Index Array(array=w577) -> (element #1=w576:string, element #2=w575:string)  [unwired: 2 in]
                  n222 = Search and Replace String(replace all?=TRUE ("replace all? (F)"), input string=w580, search string=w576, replace string=w575) -> (result string=w578:string)  [unwired: 4 in, 3 out]
                }
                n223 = for {
                  tunnel: w560 -> [w565] mode=indexing
                  tunnel: [w564] -> w559 mode=indexing
                  tunnel: w558 -> [w563]
                  n224 = for {
                    tunnel: w565 -> [w568] mode=indexing
                    tunnel: [w567] -> w564 mode=indexing
                    tunnel: w563 -> [w566]
                    n225 = for {
                      shift-right: [w572] -> w567
                      shift-left: w568 -> [w574]
                      tunnel: w566 -> [w571] mode=indexing
                      n226 = Index Array(array=w571) -> (element #1=w570:string, element #2=w569:string)  [unwired: 2 in]
                      n227 = Search and Replace String(replace all?=TRUE ("replace all? (F)"), input string=w574, search string=w570, replace string=w569) -> (result string=w572:string)  [unwired: 4 in, 3 out]
                    }
                  }
                }
                n228 = in-place-cluster #1("Worksheet"=w561, "Cells"=w559) -> (w555:cluster{"Worksheet":string, "Cells":string[][]})
              }
            }
            n229 = Bundle By Name(cluster=w554, "Worksheets"=w549) -> (w550:T2)
          }
          frame "Return Worksheets" {
            n230 = Unbundle By Name(w585) -> ("Worksheets"=w584:T1)
            n231 = case "Truncate?" shown="True" w582 {
              tunnel: w584 -> [w586 w588]
              tunnel: [w586 w587] -> w581
              frame False {
              }
              frame True {
                n232 = for {
                  tunnel: w588 -> [w590] mode=indexing
                  tunnel: [w589] -> w587 mode=indexing
                  n233 = in-place {
                    # "0: Rows\n1: Cols"
                    # "Remove empty rows/columns from end"
                    n234 = in-place-cluster #2(w590) -> ("Cells"=w593:string[][])
                    n235 = Array Size(array=w593) -> (size(s)=w599:i32[])
                    n236 = Index Array(array=w599) -> (element #1=w595:i32, element #2=w596:i32)  [unwired: 2 in]
                    n237 = for {
                      N: w595 -> [w617]
                      tunnel: w593 -> [w618]
                      tunnel: w596 -> [w613]
                      tunnel: [w612] -> w598
                      i -> [w616]
                      stop <- w614 continue-if-true
                      # "Find last non-empty row"
                      n238 = Decrement(x=w617) -> (x-1=w615:i32)
                      n239 = Subtract(x=w615, y=w616) -> (x-y=w612:i32)
                      n240 = for {
                        N: w613 -> [_]
                        tunnel: w618 -> [w623]
                        tunnel: w612 -> [w622]
                        tunnel: [w619] -> w614
                        i -> [w621]
                        stop <- w619 continue-if-true
                        n241 = Index Array(array=w623, index (row)=w622, index (col)=w621) -> (element=w620:string)
                        n242 = Empty String/Path?(string/path=w620) -> (empty?=w619:bool)
                      }
                    }
                    n243 = Increment(x=w598) -> (x+1=w591:i32)
                    n244 = for {
                      N: w596 -> [w605]
                      tunnel: w593 -> [w606]
                      tunnel: [w601] -> w597
                      tunnel: w591 -> [w600]
                      i -> [w604]
                      stop <- w602 continue-if-true
                      # "Find last non-empty column"
                      n245 = Decrement(x=w605) -> (x-1=w603:i32)
                      n246 = Subtract(x=w603, y=w604) -> (x-y=w601:i32)
                      n247 = for {
                        N: w600 -> [_]
                        tunnel: w606 -> [w611]
                        tunnel: w601 -> [w607]
                        tunnel: [w609] -> w602
                        i -> [w608]
                        stop <- w609 continue-if-true
                        n248 = Index Array(array=w611, index (row)=w608, index (col)=w607) -> (element=w610:string)
                        n249 = Empty String/Path?(string/path=w610) -> (empty?=w609:bool)
                      }
                    }
                    n250 = Increment(x=w597) -> (x+1=w594:i32)
                    n251 = Array Subset(array=w593, length (row)=w591, length (col)=w594) -> (w592:string[][])  [unwired: 2 in]
                    n252 = in-place-cluster #2("Cells"=w592) -> (w589:cluster{"Worksheet":string, "Cells":string[][]})
                  }
                }
              }
            }
          }
        }
        n253 = Empty String/Path?(string/path=w18) -> (empty?=w17:bool)
        n254 = Or(x=w17, y=w20) -> (x .or. y?=w19:bool)
      }
    }
    frame Error {
    }
  }
  "error out" <- w3
  "Worksheets" <- w2
  "Path out" <- "Path in (xlsx,tsv,txt,csv,xml)"
